vi "Clusters.vi"() -> ()   [LabVIEW 2020]
panel:
  out "output cluster 2":T1
  in  "Trama IOT":string
  in  "Salidas digitalaes s71200":bool[](array[boolean])
  in  "SELECTOR":u16(knob) scale=0.0..10.0
  in  "Termocupla":dbl(slide) scale=0.0..100.0
  out "output cluster":T2
  in  "Meter":dbl(knob) scale=0.0..60.0
  out "Send Data":string
  out "Pesaje":u32
  out "Variador de Velocidad":dbl
  out "Start":bool
  in  "Pesadora de Pescado":T2 {"Variador de Velocidad" scale=0.0..60.0}
  # "Clusters"
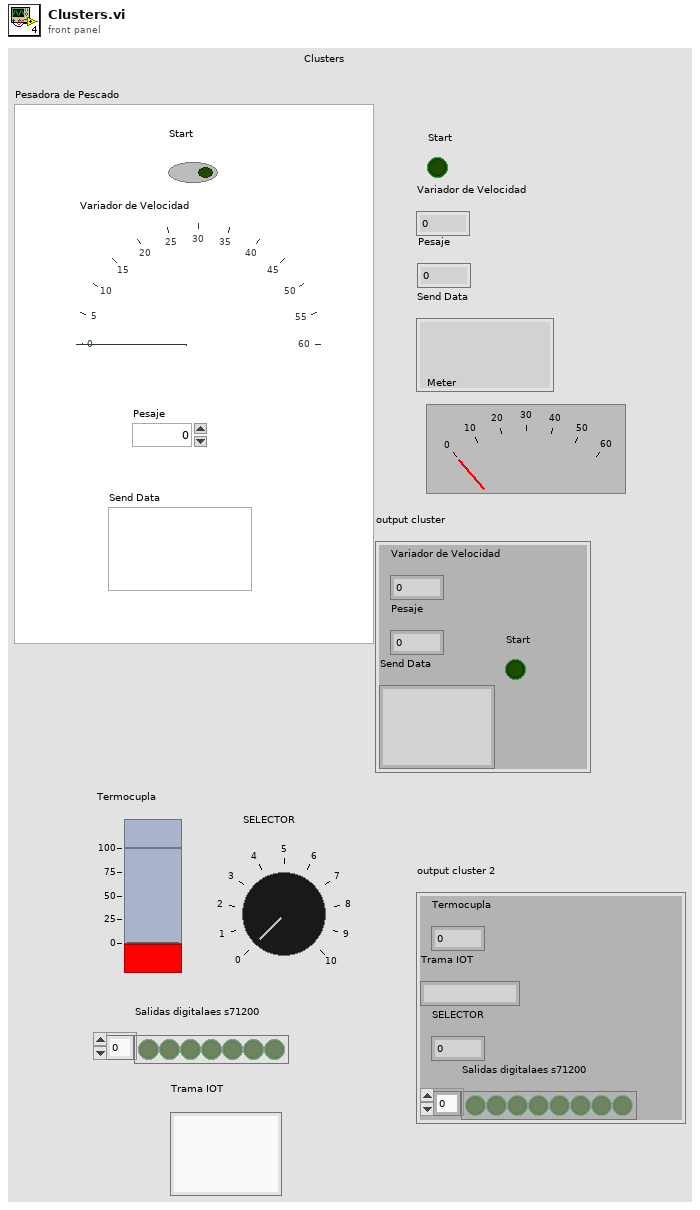
[diagram p1: front panel]
types:
  T1 = cluster{"Termocupla":dbl, "Trama IOT":string, "SELECTOR":u16, "Salidas digitalaes s71200":bool[]}
  T2 = cluster{"Variador de Velocidad":dbl, "Pesaje":u32, "Send Data":string, "Start":bool}
  T3 = cluster{"Data_Microcontrolador":cluster{"ADC":dbl[], "ON/OFF":bool, "UART":string}, "Data_PLC":cluster{"Direccion IP":string, "Puerto":i32, "Pinzadora":i32[], "Variadores":dbl[]}, "TRAMA_IOT":cluster{"Dominio":string, "Puerto TCP":i32, "Token":string, "Device":string}, "Alarmas":cluster{"alarma s71200":bool[]}}
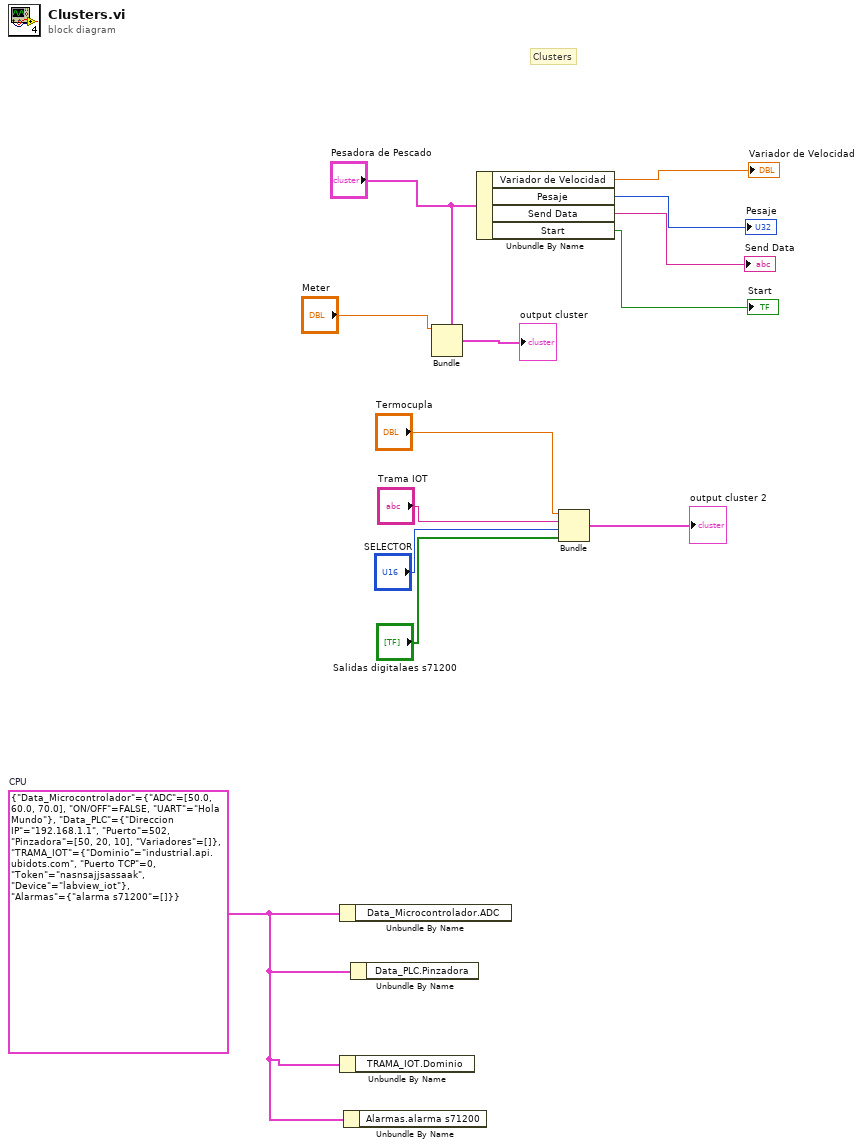
[diagram p0: block diagram]
diagram:
  w1 = T3 {"Data_Microcontrolador"={"ADC"=[50.0, 60.0, 70.0], "ON/OFF"=FALSE, "UART"="Hola Mundo"}, "Data_PLC"={"Direccion IP"="192.168.1.1", "Puerto"=502, "Pinzadora"=[50, 20, 10], "Variadores"=[]}, "TRAMA_IOT"={"Dominio"="industrial.api.ubidots.com", "Puerto TCP"=0, "Token"="nasnsajjsassaak", "Device"="labview_iot"}, "Alarmas"={"alarma s71200"=[]}}  # CPU
  # "Clusters"
  n1 = Unbundle By Name(w1) -> ()  [unwired: 1 out]
  n2 = Unbundle By Name(w1) -> ()  [unwired: 1 out]
  n3 = Unbundle By Name(w1) -> ()  [unwired: 1 out]
  n4 = Unbundle By Name(w1) -> ()  [unwired: 1 out]
  n5 = Bundle(cluster="Pesadora de Pescado", "Variador de Velocidad"="Meter") -> (→"output cluster":T2)  [unwired: 3 in]
  n6 = Unbundle By Name("Pesadora de Pescado") -> ("Variador de Velocidad"=→"Variador de Velocidad":dbl, "Pesaje"=→"Pesaje":u32, "Send Data"=→"Send Data":string, "Start"=→"Start":bool)
  n7 = Bundle("Termocupla"="Termocupla", "Trama IOT"="Trama IOT", "SELECTOR"="SELECTOR", "Salidas digitalaes s71200"="Salidas digitalaes s71200") -> (→"output cluster 2":T1)  [unwired: 1 in]
